vi "RandNumberRange.vi"(1 "Max":dbl, 2 "Min":dbl) -> (0 "Value":dbl)   [LabVIEW 2011]
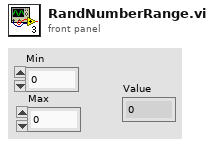
[diagram p1: front panel]
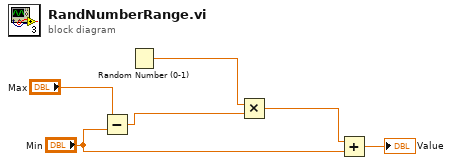
[diagram p0: block diagram]
diagram:
  n1 = Subtract(x="Max", y="Min") -> (x-y=w4:dbl)
  n2 = Random Number (0-1)() -> (number: 0 to 1=w5:dbl)
  n3 = Multiply(x=w5, y=w4) -> (x*y=w3:dbl)
  n4 = Add(x=w3, y="Min") -> (x+y=→"Value":dbl)
